vi "test_distributeHorizontalCentersShouldWork.vi"(11 "Test Case In":refnum<class "DistributeCentersTests.lvclass">) -> (0 "error out":errorcluster, 3 "Test Case Out":refnum<class "DistributeCentersTests.lvclass">)   [LabVIEW 2023, in "DistributeCentersTests.lvclass"]
uses:
  DistributeCentersTests.lvclass
  source/Ctrls/alignment.ctl
  <vilib>/Astemes/LUnit/Test Case.lvclass/Test Case.ctl
  source/Misc/getBoundsRect.vi
  <vilib>/Astemes/LUnit/Core/LUnit Test Case/Private/Append Fail Result.vi
  <vilib>/Astemes/LUnit/Core/LUnit Test Case/Private/Append Pass Result.vi
  source/Misc/processUseControlBodyOnlyFlag_start.vi
  source/Misc/processUseControlBodyOnlyFlag_end.vi
  <vilib>/Astemes/LUnit/Core/LUnit Test Case/Private/Run In UI.vi
  <vilib>/Utility/error.llb/Clear Errors.vi
  source/Misc/hideCaption&Label.vi
  source/Misc/setCaption&LabelVisibility.vi
  DistributeCentersTests.lvclass/DistributeCentersTests.ctl
  <vilib>/Astemes/LUnit/Test Case.lvclass
  C:/Program Files (x86)/National Instruments/LabVIEW 2023/vi.lib/Astemes/LUnit/Test Case.lvclass
  C:/Program Files (x86)/National Instruments/LabVIEW 2023/vi.lib/Astemes/LUnit/LUnit Runnable.lvclass
  C:/projects/TLC_Geometry/tests/DistributeCentersTests/DistributeCentersTests.lvclass
panel:
  in  "Numeric_topRight":dbl
  in  "btn":bool
  in  "firstItem_topLeft":string
  in  "String":string
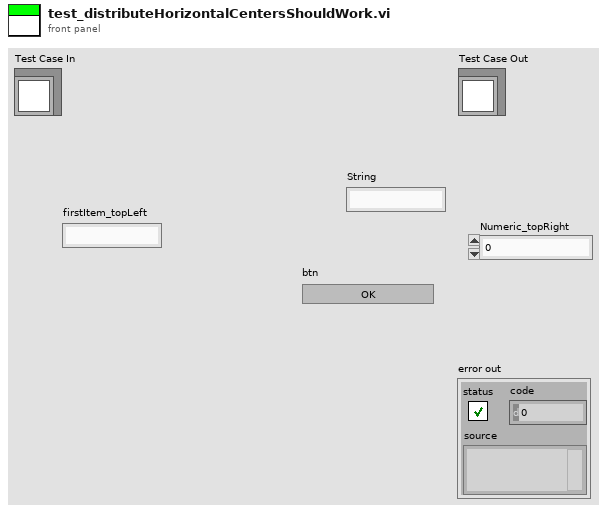
[diagram p1: front panel]
types:
  T1 = typedef "alignment.ctl" = enum16{"None", "AlignTop", "AlignBottom", "AlignHorizontalCenters", "AlignLeft", "AlignRight", "AlignVerticalCenters"}
  T2 = typedef "LVPositionTypeDef.ctl" = cluster{"Left":i32, "Top":i32}
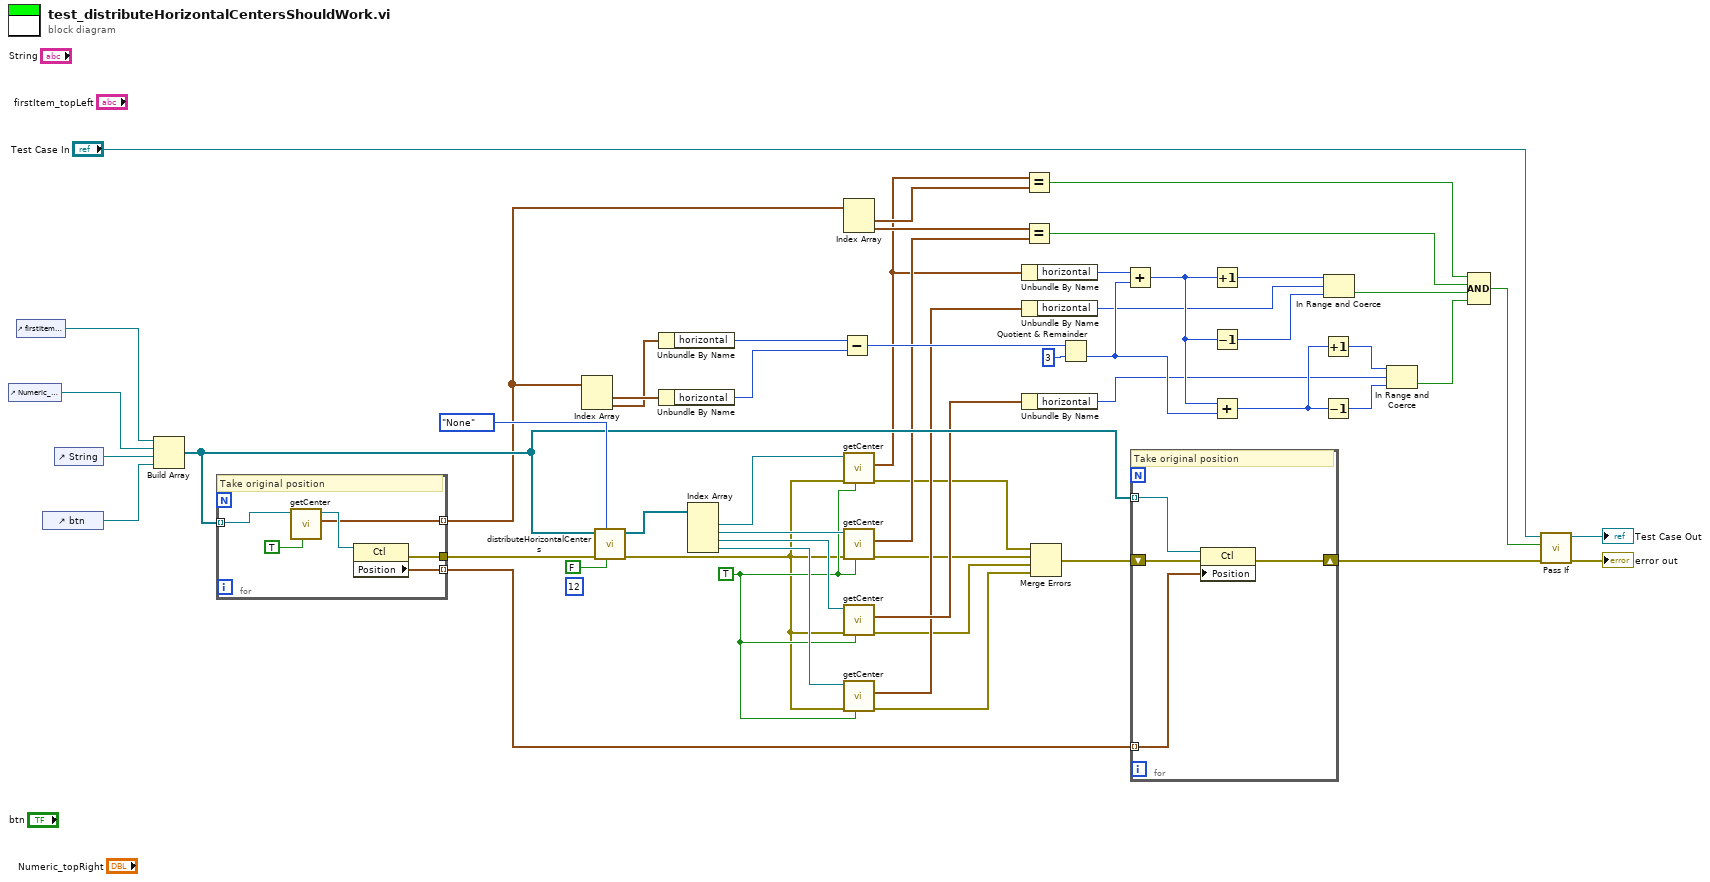
[diagram p0: block diagram]
diagram:
  w18 = TRUE ("useControlBodyOnly")
  (unwired) u16 12 ("spacing")
  n1 = control-ref of="Numeric_topRight"() -> (w46:refnum<vi>)
  n2 = control-ref of="firstItem_topLeft"() -> (w47:refnum<vi>)
  n3 = control-ref of="btn"() -> (w43:refnum<vi>)
  n4 = control-ref of="String"() -> (w44:refnum<vi>)
  n5 = Build Array(w47, w46, w44, w43) -> (w45:refnum<vi>[])
  n6 = for {
    tunnel: w45 -> [w59] mode=indexing
    tunnel: [w58] -> w35 mode=indexing
    tunnel: [w57] -> w50
    tunnel: [w55] -> w29 mode=indexing
    # "Take original position"
    n7 = call "getCenter.vi"("useControlBodyOnly"=TRUE, "ref"=w59) -> ("center"=w55:cluster{"horizontal":i32, "vertical":i32}, "ref(dup)"=w56:refnum<vi>)  [unwired: 7 in, 1 out]
    n8 = property class="Ctl"(reference=w56) -> (error out=w57:errorcluster, "Position"=w58:T2)  [unwired: 1 in, 1 out]
  }
  n9 = Index Array(array=w29) -> (element #1=w42:cluster{"horizontal":i32, "vertical":i32}, element #2=w41:cluster{"horizontal":i32, "vertical":i32})  [unwired: 2 in]
  n10 = call "distributeHorizontalCenters.vi"("useControlBodyOnly"=FALSE, "verticalAlignment"=alignment."None", "error in (no error)"=w50, "refs"=w45) -> ("error out"=w17:errorcluster, "refs(dup)"=w36:refnum<vi>[])  [unwired: 6 in]
  n11 = Unbundle By Name(w41) -> ("horizontal"=w39:i32)
  n12 = Unbundle By Name(w42) -> ("horizontal"=w40:i32)
  n13 = Index Array(array=w36) -> (element #1=w30:refnum<vi>, element #2=w28:refnum<vi>, element #3=w32:refnum<vi>, element #4=w31:refnum<vi>)  [unwired: 4 in]
  n14 = Subtract(x=w39, y=w40) -> (x-y=w38:i32)
  n15 = Index Array(array=w29) -> (element #1=w34:cluster{"horizontal":i32, "vertical":i32}, element #2=w33:cluster{"horizontal":i32, "vertical":i32})  [unwired: 2 in]
  n16 = call "getCenter.vi"("useControlBodyOnly"=w18, "error in (no error)"=w17, "ref"=w30) -> ("error out"=w16:errorcluster, "center"=w26:cluster{"horizontal":i32, "vertical":i32})  [unwired: 6 in, 1 out]
  n17 = call "getCenter.vi"("useControlBodyOnly"=w18, "error in (no error)"=w17, "ref"=w28) -> ("error out"=w15:errorcluster, "center"=w27:cluster{"horizontal":i32, "vertical":i32})  [unwired: 6 in, 1 out]
  n18 = call "getCenter.vi"("useControlBodyOnly"=w18, "error in (no error)"=w17, "ref"=w32) -> ("error out"=w14:errorcluster, "center"=w24:cluster{"horizontal":i32, "vertical":i32})  [unwired: 6 in, 1 out]
  n19 = call "getCenter.vi"("useControlBodyOnly"=w18, "error in (no error)"=w17, "ref"=w31) -> ("error out"=w13:errorcluster, "center"=w23:cluster{"horizontal":i32, "vertical":i32})  [unwired: 6 in, 1 out]
  n20 = Unbundle By Name(w26) -> ("horizontal"=w25:i32)
  n21 = Unbundle By Name(w23) -> ("horizontal"=w2:i32)
  n22 = Unbundle By Name(w24) -> ("horizontal"=w1:i32)
  n23 = Equal?(x=w26, y=w34) -> (x = y?=w21:bool)
  n24 = Equal?(x=w33, y=w27) -> (x = y?=w20:bool)
  n25 = Merge Errors(w16, w15, w14, w13) -> (w12:errorcluster)
  n26 = Quotient & Remainder(x=w38, y=3) -> (floor(x/y)=w22:i32)  [unwired: 1 out]
  n27 = Add(x=w25, y=w22) -> (x+y=w4:i32)
  n28 = for {
    tunnel: w45 -> [w63] mode=indexing
    tunnel: w35 -> [w62] mode=indexing
    shift-right: [w61] -> w11
    shift-left: w12 -> [w60]
    # "Take original position"
    n29 = property class="Ctl"(reference=w63, error in=w60, "Position"=w62) -> (error out=w61:errorcluster)  [unwired: 1 out]
  }
  n30 = Increment(x=w4) -> (x+1=w6:i32)
  n31 = Decrement(x=w4) -> (x-1=w5:i32)
  n32 = Add(x=w4, y=w22) -> (x+y=w10:i32)
  n33 = Increment(x=w10) -> (x+1=w9:i32)
  n34 = Decrement(x=w10) -> (x-1=w8:i32)
  n35 = In Range and Coerce(upper limit=w6, x=w2, lower limit=w5) -> (In Range?=w3:bool)  [unwired: 1 out]
  n36 = In Range and Coerce(upper limit=w9, x=w1, lower limit=w8) -> (In Range?=w7:bool)  [unwired: 1 out]
  n37 = Compound Arithmetic op=AND(w21, w20, w3, w7) -> (w19:bool)
  n38 = call <vilib>:"Pass If.vi"("error in (no error)"=w11, "Pass?"=w19, "LUnit Test Case In"="Test Case In") -> ("error out"=→"error out":errorcluster, "LUnit Test Case Out"=→"Test Case Out":refnum<class "DistributeCentersTests.lvclass">)  [unwired: 7 in]
